vi "Check_Subtrack_Length-2.vi"(2 "[IN] Subtrack":T1, 3 "[IN] Minimal Sub\ntrack Length":i32) -> (0 "[OUT] Subtrack":T1)   [LabVIEW 2013]
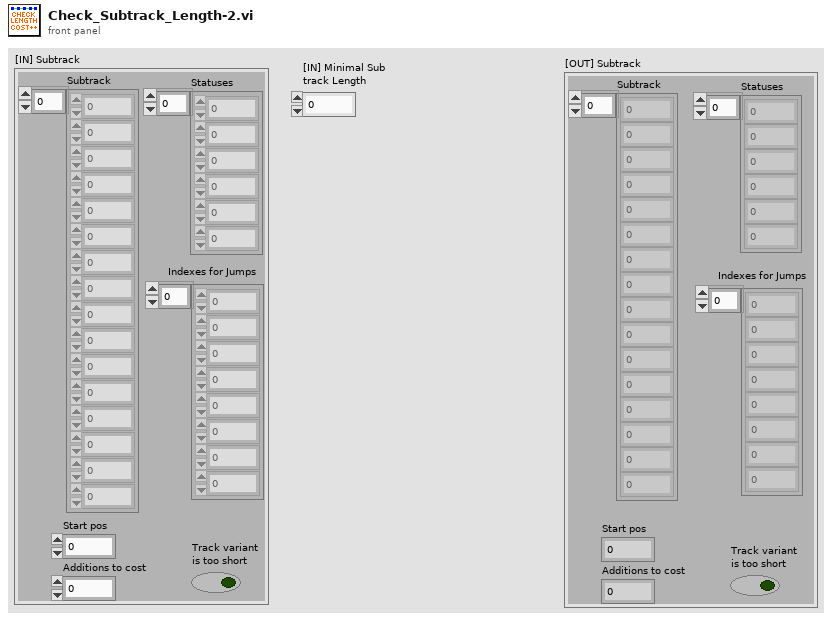
[diagram p1: front panel]
types:
  T1 = cluster{"Subtrack":dbl[], "Statuses":i16[], "Start pos":i32, "Additions to cost":i32, "Track variant \nis too short":bool, "Indexes for Jumps":i32[]}
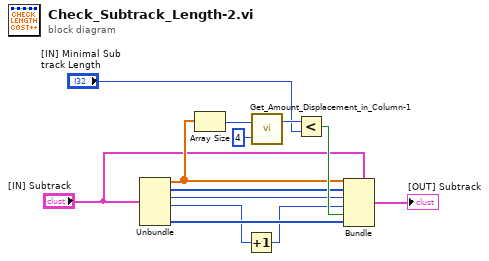
[diagram p0: block diagram]
diagram:
  n1 = Unbundle("[IN] Subtrack") -> ("Subtrack"=w8:dbl[], "Statuses"=w9:i16[], "Start pos"=w7:i32, "Additions to cost"=w2:i32, "Indexes for Jumps"=w6:i32[])  [unwired: 1 out]
  n2 = Array Size(array=w8) -> (size(s)=w13:i32)
  n3 = Increment(x=w2) -> (x+1=w1:i32)
  n4 = call "Get_Amount_Displacement_in_Column-1.vi"("multiplier"=4, "# Rows"=w13) -> ("Displ amount"=w12:i32)  [unwired: 1 out]
  n5 = Less?(x=w12, y="[IN] Minimal Sub\ntrack Length") -> (x < y?=w10:bool)
  n6 = Bundle(cluster="[IN] Subtrack", "Subtrack"=w8, "Statuses"=w9, "Start pos"=w7, "Additions to cost"=w1, "Track variant \nis too short"=w10, "Indexes for Jumps"=w6) -> (→"[OUT] Subtrack":T1)
